vi "OnDoubleClick.vi"(0 "XRef":T12, 1 "Point":T10, 2 "State In":T1 {"BlockNodeState"."Draw Style" items=["FunctionBlock", "ExpressVI", "Variable", "Elemental I/O", "32x32 Icon", "FunctionBlockCompact"]; "BlockNodeState"."Terminal Data"."Terminal Flags" format="%.0b"}) -> (14 "Reply":T8, 15 "State Out":T1 {"BlockNodeState"."Draw Style" items=["FunctionBlock", "ExpressVI", "Variable", "Elemental I/O", "32x32 Icon", "FunctionBlockCompact"]; "BlockNodeState"."Terminal Data"."Terminal Flags" format="%.0b"})   [LabVIEW 2020, in "NI_ExpressFull.lvlib" / "ExpressSpectralMeasurementsBlockNode.xnode"]
uses:
  <vilib>/express/express analysis/Spectral/XNode/ExpressSpectralMeasurementsBlockNode.xnode
  <vilib>/XNodeSupport/XNodeXNodeRef.ctl
  <vilib>/XNodeSupport/NI_XNodeSupport.lvlib
  <vilib>/XNodeSupport/XNodeInt.ctl
  <vilib>/XNodeSupport/XNodePoint.ctl
  <vilib>/XNodeSupport/XNodeStringArray.ctl
  <vilib>/XNodeSupport/XNodeString.ctl
  <vilib>/picture/picture.llb/imagedata.ctl
  <vilib>/BlockNodeSupport/BlockNodeState.ctl
  <vilib>/express/express analysis/Spectral/XNode/State.ctl
  <vilib>/express/express shared/XNodes/controls/ExpressState.ctl
  <vilib>/BlockNodeSupport/TerminalData.ctl
  <vilib>/XNodeSupport/XNodeType.ctl
  <vilib>/express/express shared/XNodes/controls/ExpressTerminalInfo.ctl
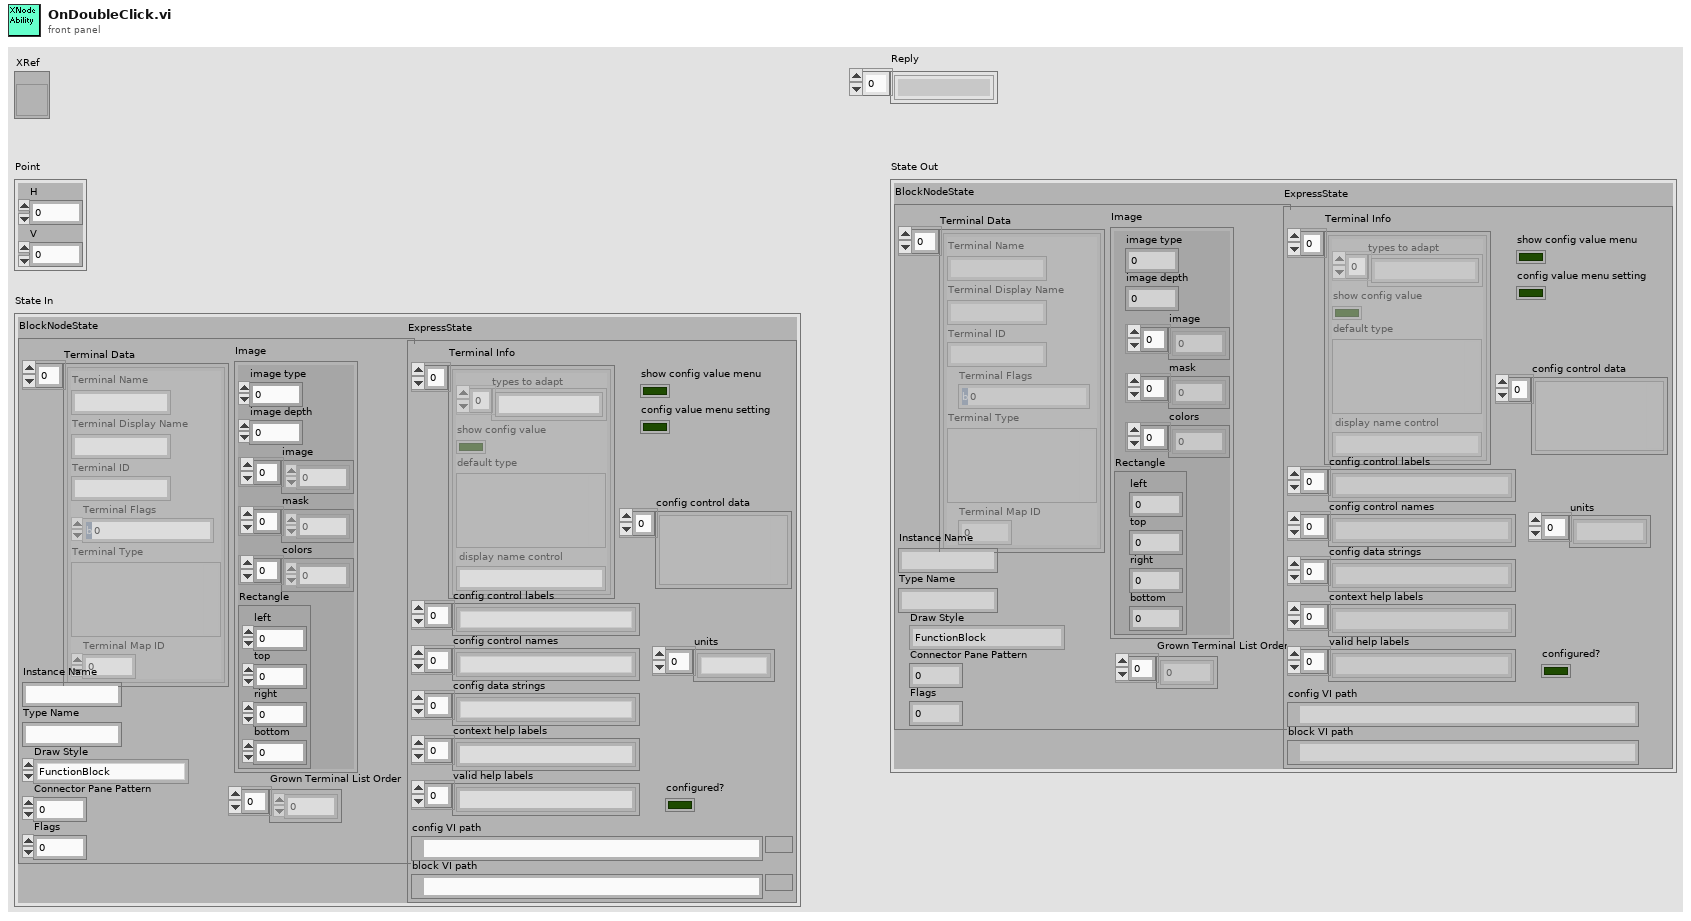
[diagram p1: front panel]
types:
  T1 = typedef "NI_ExpressFull.lvlib/ExpressSpectralMeasurementsBlockNode.xnode/State.ctl" = cluster{"BlockNodeState":T2, "ExpressState":T5}
  T2 = typedef "BlockNodeState.ctl" = cluster{"Terminal Data":T3[], "Instance Name":string, "Type Name":string, "Draw Style":i32, "Connector Pane Pattern":i32, "Flags":i32, "Grown Terminal List Order":i32[], "Image":T4}
  T3 = typedef "TerminalData.ctl" = cluster{"Terminal Name":string, "Terminal Display Name":string, "Terminal ID":string, "Terminal Flags":i32, "Terminal Type":variant, "Terminal Map ID":i32}
  T4 = typedef "imagedata.ctl" = cluster{"image type":i32, "image depth":i32, "image":u8[], "mask":u8[], "colors":u32[], "Rectangle":cluster{"left":i16, "top":i16, "right":i16, "bottom":i16}}
  T5 = typedef "ExpressState.ctl" = cluster{"Terminal Info":T6, "config control names":string[], "config data strings":string[], "config control data":variant[], "units":string[], "configured?":bool, "config VI path":path, "block VI path":path, "config control labels":string[], "show config value menu":bool, "config value menu setting":bool, "context help labels":string[], "valid help labels":string[]}
  T6 = typedef "ExpressTerminalInfo.ctl" = cluster{"types to adapt":string[], "show config value":bool, "default type":T7, "display name control":string}[]
  T7 = typedef "NI_XNodeSupport.lvlib/XNodeType.ctl" = variant
  T8 = typedef "NI_XNodeSupport.lvlib/XNodeStringArray.ctl" = T9[]
  T9 = typedef "NI_XNodeSupport.lvlib/XNodeString.ctl" = string
  T10 = typedef "NI_XNodeSupport.lvlib/XNodePoint.ctl" = cluster{"H":T11, "V":T11}
  T11 = typedef "NI_XNodeSupport.lvlib/XNodeInt.ctl" = i32
  T12 = typedef "NI_XNodeSupport.lvlib/XNodeXNodeRef.ctl" = refnum<vi>
  T13 = typedef "ExpressBlockNodeState.ctl" = cluster{"BlockNodeState":T2, "ExpressState":T5}
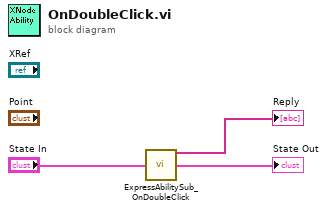
[diagram p0: block diagram]
diagram:
  n1 = call <vilib>:"ExpressAbilitySub_OnDoubleClick.vi"("ExpressBlockNodeState In"="State In") -> ("Reply"=→"Reply":string[], "ExpressBlockNodeState Out"=→"State Out":T13)  [unwired: 13 in]
